vi "TaskCreationEvents.vi"(8 "error in (no error)":errorcluster, 11 "DAQmx(AI) in":refnum<class "DAQmx(AI).lvclass">) -> (0 "error out":errorcluster, 3 "DAQmx(AI) out":refnum<class "DAQmx(AI).lvclass">)   [LabVIEW 2013, in "DAQmx(AI).lvclass"]
uses:
  DAQmx(AI).lvclass
  Typedefs/ScalingEvent--Cluster.ctl
  Typedefs/Scaling(MapRange)--Cluster.ctl
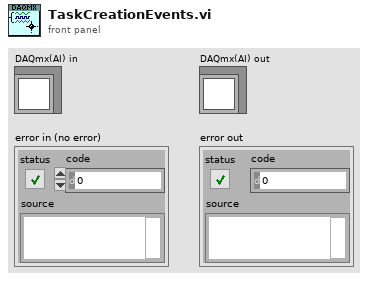
[diagram p1: front panel]
types:
  T1 = typedef "DAQmx(AI).lvclass/ScalingEvent--Cluster.ctl" = cluster{"Scale Name":string, "Units":string, "Range":T2}
  T2 = typedef "DAQmx(AI).lvclass/Scaling(MapRange)--Cluster.ctl" = cluster{"Minimum":dbl, "Maximum":dbl}
  T3 = typedef "DAQmx(AI).lvclass/PublicEvents--Cluster.ctl" = cluster{"Value Changed":refnum<user-event>, "Task Configuration":refnum<user-event>, "Scaling":refnum<user-event>}
  T4 = typedef "DAQmx(AI).lvclass/Configuration--Cluster.ctl" = cluster{"PhysChan":tag, "Period (ms)":i64, "input terminal cfg":i32, "minimum value":dbl, "maximum value":dbl, "units":T5, "task name":string}
  T5 = typedef "DAQmx(AI).lvclass/Units -- Enum.ctl" = enum16{"Volts", "Amps", "Deg F", "Deg C", "Deg R", "Kelvins", "Strain", "Ohms", "Hz", "Seconds", "Meters", "Inches", "Degrees", "Radians", "Ticks", "g", "m/s^2", "m/s", "in/s", "Pascals", "Newtons", "Pounds", "kgf", "psi", "bar", "Nm", "oz-in", "lb-in", "lb-ft", "Volts/Volt", "mVolts/Volt", "From TEDS"}
  T6 = typedef "DAQmx(AI).lvclass/Scaling--Cluster.ctl" = cluster{"Scale Name":string, "Scale Type":T7, "Scaled Units":string, "Linear":T8, "Map Range":T2, "Polynomial":T9, "Table":T10}
  T7 = typedef "DAQmx(AI).lvclass/ScalingType--Enum.ctl" = enum16{"No scaling", "Linear", "Map Range", "Polynomial", "Table"}
  T8 = typedef "DAQmx(AI).lvclass/Scaling(Linear)--Cluster.ctl" = cluster{"Slope":dbl, "Intercept":dbl}
  T9 = typedef "DAQmx(AI).lvclass/Scaling(Polynomial)--Cluster.ctl" = cluster{"forward coeff":dbl[], "reverse coeff":dbl[]}
  T10 = typedef "DAQmx(AI).lvclass/Scaling(Table)--Cluster.ctl" = cluster{"scaled values":dbl[], "pres-scaled values":dbl[]}
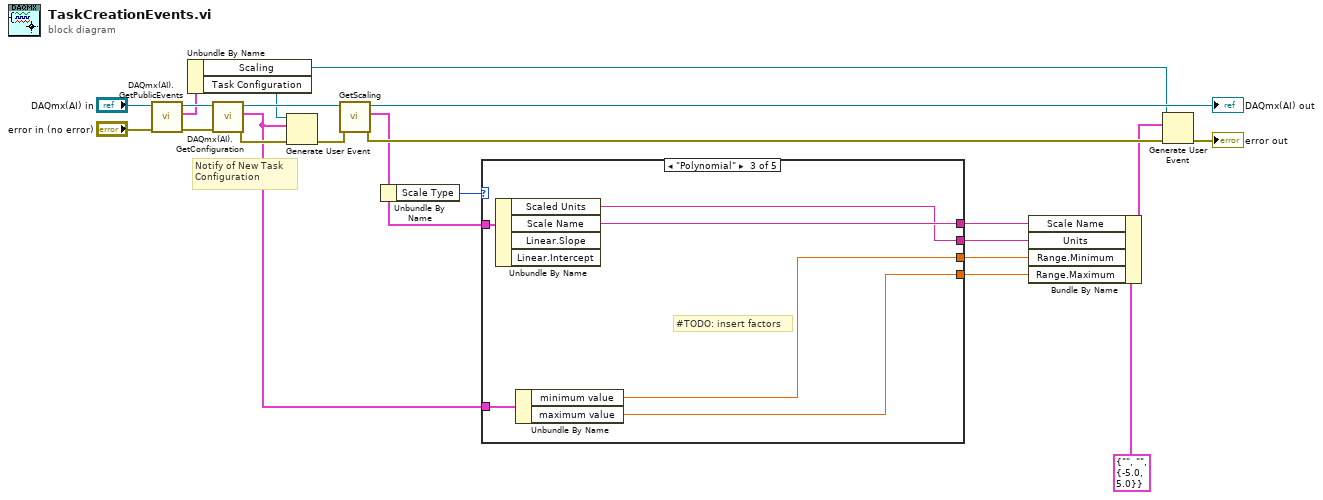
[diagram p0: block diagram]
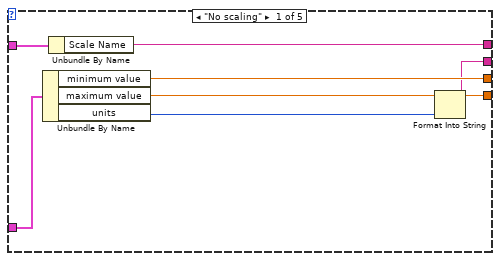
[diagram p2: hidden frame]
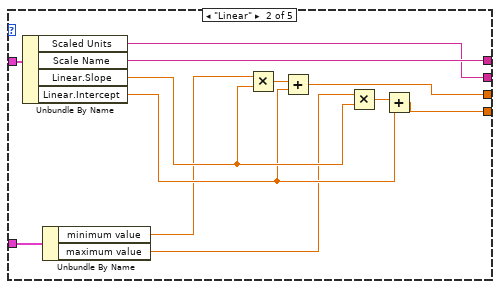
[diagram p3: hidden frame]
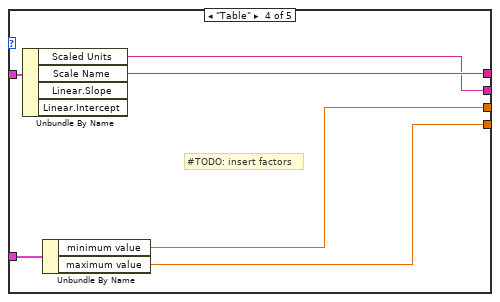
[diagram p4: hidden frame]
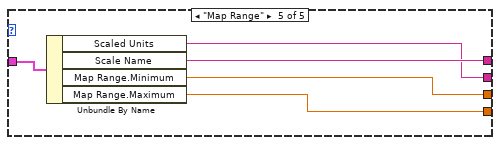
[diagram p5: hidden frame]
diagram:
  # "Notify of New Task\nConfiguration"
  n1 = call "DAQmx(AI).GetPublicEvents.vi"("error in (no error)"="error in (no error)", "Subsystem"="DAQmx(AI) in") -> ("error out"=w15:errorcluster, "DAQmx(AI) Public Events"=w11:T3, "Subsystem out"=w14:refnum<class "DAQmx(AI).lvclass">)  [unwired: 7 in]
  n2 = Unbundle By Name(w11) -> ("Scaling"=w18:refnum<user-event>, "Task Configuration"=w10:refnum<user-event>)
  n3 = call "DAQmx(AI).GetConfiguration.vi"("error in (no error)"=w15, "Subsystem"=w14) -> ("error out"=w16:errorcluster, "Configuration"=w4:T4, "Subsystem out"=w19:refnum<class "DAQmx(AI).lvclass">)  [unwired: 7 in]
  n4 = Generate User Event(user event=w10, event data cluster=w4, error in=w16) -> (error out=w22:errorcluster)  [unwired: 1 in, 1 out]
  n5 = call "GetScaling.vi"("error in (no error)"=w22, "Subsystem"=w19) -> ("error out"=w21:errorcluster, "Scaling"=w5:T6, "Subsystem out"=→"DAQmx(AI) out":refnum<class "DAQmx(AI).lvclass">)  [unwired: 6 in, 1 out]
  n6 = Unbundle By Name(w5) -> ("Scale Type"=w6:T7)
  n7 = case shown="\"Polynomial\"" w6 {
    tunnel: [w29 w41 w47 w53 w58] -> w8
    tunnel: w5 -> [w28 w40 w46 w52 w57]
    tunnel: w4 -> [w27 w39 w45 w51 _]
    tunnel: [w26 w31 w42 w48 w55] -> w3
    tunnel: [w24 w38 w44 w50 w56] -> w2
    tunnel: [w23 w30 w43 w49 w54] -> w1
    frame "No scaling" {
      n8 = Unbundle By Name(w27) -> ("minimum value"=w26:dbl, "maximum value"=w23:dbl, "units"=w25:T5)
      n9 = Unbundle By Name(w28) -> ("Scale Name"=w29:string)
      n10 = Format Into String(w25) -> (resulting string=w24:string)  [unwired: 3 in, 1 out]
    }
    frame "Linear" {
      n11 = Unbundle By Name(w40) -> ("Scaled Units"=w38:string, "Scale Name"=w41:string, "Linear.Slope"=w35:dbl, "Linear.Intercept"=w34:dbl)
      n12 = Unbundle By Name(w39) -> ("minimum value"=w33:dbl, "maximum value"=w32:dbl)
      n13 = Multiply(x=w33, y=w35) -> (x*y=w37:dbl)
      n14 = Add(x=w37, y=w34) -> (x+y=w31:dbl)
      n15 = Multiply(x=w32, y=w35) -> (x*y=w36:dbl)
      n16 = Add(x=w36, y=w34) -> (x+y=w30:dbl)
    }
    frame "Polynomial" {
      # "#TODO: insert factors"
      n17 = Unbundle By Name(w46) -> ("Scaled Units"=w44:string, "Scale Name"=w47:string)  [unwired: 2 out]
      n18 = Unbundle By Name(w45) -> ("minimum value"=w42:dbl, "maximum value"=w43:dbl)
    }
    frame "Table" {
      # "#TODO: insert factors"
      n19 = Unbundle By Name(w52) -> ("Scaled Units"=w50:string, "Scale Name"=w53:string)  [unwired: 2 out]
      n20 = Unbundle By Name(w51) -> ("minimum value"=w48:dbl, "maximum value"=w49:dbl)
    }
    frame "Map Range" {
      n21 = Unbundle By Name(w57) -> ("Scaled Units"=w56:string, "Scale Name"=w58:string, "Map Range.Minimum"=w55:dbl, "Map Range.Maximum"=w54:dbl)
    }
  }
  n22 = Bundle By Name(cluster=T1 {"Scale Name"="", "Units"="", "Range"={"Minimum"=-5.0, "Maximum"=5.0}} ("Scaling Event"), "Scale Name"=w8, "Units"=w2, "Range.Minimum"=w3, "Range.Maximum"=w1) -> (w7:T1)
  n23 = Generate User Event(user event=w18, event data cluster=w7, error in=w21) -> (error out=→"error out":errorcluster)  [unwired: 1 in, 1 out]
